vi "Create from Known Hosts.vi"(8 "Error In":errorcluster, 11 "Known Hosts In":refnum<class "Known Hosts.lvclass">) -> (0 "Error Out":errorcluster, 2 "Known Host":refnum<class "Known Host.lvclass">, 3 "Known Hosts Out":refnum<class "Known Hosts.lvclass">)   [LabVIEW 2021, in "Field_RnD_Services_LIBSSH2_Toolkit.lvlib" / "Known Host.lvclass"]
doc: "Passes through the Known Hosts object but obtains the SSH context for the Known Hosts object to create a new Known Host object."
uses:
  Known Host.lvclass
  Known Hosts/Known Hosts.lvclass
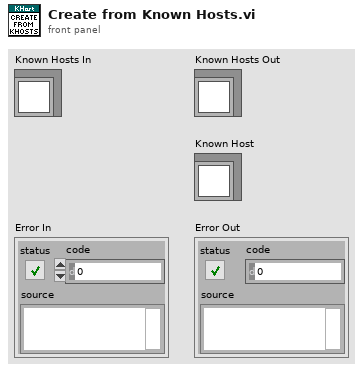
[diagram p1: front panel]
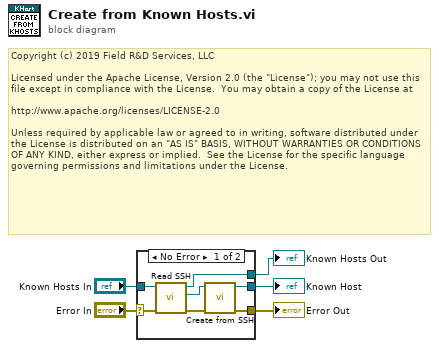
[diagram p0: block diagram]
diagram:
  # "Copyright (c) 2019 Field R&D Services, LLC\n\nLicensed under the Apache License, Version 2.0 (the \"License\"); you may not use this file except in compliance with the License.  You may obtain a copy of the License at\n\nhttp://www.apache.org/licenses/LICENSE-2.0\n\nUnless required by applicable law or agreed to in writing, software distributed under the License is distributed on an \"AS IS\" BASIS, WITHOUT WARRANTIES OR CONDITIONS OF ANY KIND, either express or implied.  See the License for the specific language governing permissions and limitations under the License."
  n1 = case shown="No Error" "Error In" {
    selector: "Error In" -> [w11 w14]
    tunnel: [w8 w14] -> w4
    tunnel: [w7 _] -> w3
    tunnel: "Known Hosts In" -> [w12 w13]
    tunnel: [w6 w13] -> w1
    frame No Error {
      n2 = call "Read SSH.vi"("Error In"=w11, "Known Hosts In"=w12) -> ("Error Out"=w9:errorcluster, "SSH"=w10:refnum<class "SSH.lvclass">, "Known Hosts Out"=w6:refnum<class "Known Hosts.lvclass">)  [unwired: 7 in]
      n3 = call "Create from SSH.vi"("Error In"=w9, "SSH"=w10) -> ("Error Out"=w8:errorcluster, "Known Host"=w7:refnum<class "Known Host.lvclass">)  [unwired: 8 in]
    }
    frame Error {
    }
  }
  "Error Out" <- w4
  "Known Host" <- w3
  "Known Hosts Out" <- w1
